vi "I2C_write.vi"(8 "Min time SCL Low":u32 caption="Low", 9 "Min time SCL High":u32 caption="High", 11 "Data":u8[](array[numeric])) -> ()   [LabVIEW 2019]
uses:
  <vilib>/rvi/Emulation/niFpgaGetClockAttributes.vi
  <vilib>/rvi/Emulation/niFpgaSctlEmulationGetInTimedLoop.vi
  <vilib>/rvi/Emulation/niFpgaEmulationReportErrorSimple.vi
  <vilib>/rvi/eio/common/nirviEmuTemplateMethod_errors.vi
  <vilib>/rvi/Emulation/niFpgaCriticalErrorInLSC.vi
  <vilib>/eio/EIONode/EIONode.xnode
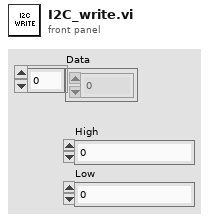
[diagram p1: front panel]
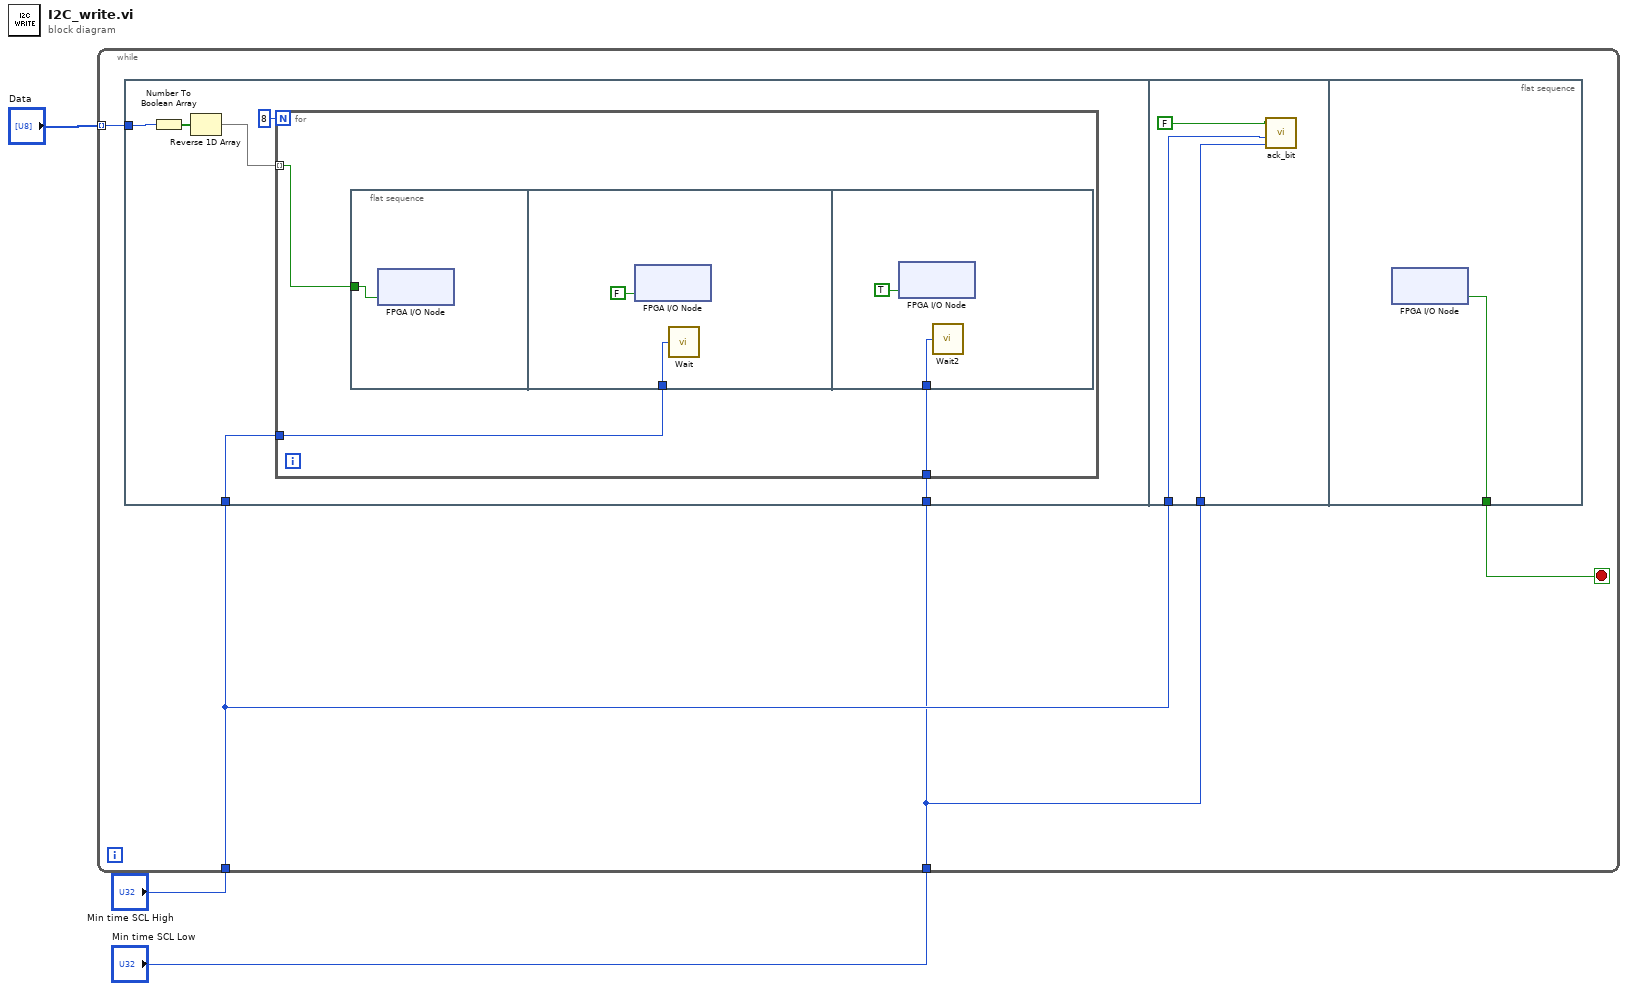
[diagram p0: block diagram]
diagram:
  n1 = while {
    tunnel: "Min time SCL High" -> [w7]
    tunnel: "Min time SCL Low" -> [w6]
    tunnel: "Data" -> [w5] mode=indexing
    stop <- w4 stop-if-true
    n2 = flat-sequence {
      tunnel: w5 -> [w8]
      tunnel: w7 -> [w10]
      tunnel: w6 -> [w9]
      tunnel: w7 -> [w23]
      tunnel: w6 -> [w22]
      tunnel: [w25] -> w4
      frame #0 {
        n3 = Number To Boolean Array(number=w8) -> (Boolean array=w13:bool[])
        n4 = Reverse 1D Array(array=w13) -> (reversed array=w11:bool[])
        n5 = for {
          N: 8 -> [_]
          tunnel: w11 -> [w16] mode=indexing
          tunnel: w10 -> [w15]
          tunnel: w9 -> [w14]
          n6 = flat-sequence {
            tunnel: w16 -> [w17]
            tunnel: w15 -> [w18]
            tunnel: w14 -> [w20]
            frame #0 {
              n7 = xnode "FPGA I/O Node"("SDA"=w17) -> ()  [unwired: 1 in, 1 out]
            }
            frame #1 {
              n8 = xnode "FPGA I/O Node"("SCL"=FALSE ("ConnectorA/DIO14")) -> ()  [unwired: 1 in, 1 out]
              n9 = call "Wait"("Count(uSec)"=w18) -> ()  [unwired: 1 out]
            }
            frame #2 {
              n10 = xnode "FPGA I/O Node"("SCL"=TRUE ("ConnectorA/DIO14")) -> ()  [unwired: 1 in, 1 out]
              n11 = call "Wait2"("Count(uSec)"=w20) -> ()  [unwired: 1 out]
            }
          }
        }
      }
      frame #1 {
        n12 = call "ack_bit.vi"("Min time SCL Low"=w22, "Min Time SCL High"=w23, "ack"=FALSE ("Acknowledgement")) -> ()  [unwired: 9 in]
      }
      frame #2 {
        n13 = xnode "FPGA I/O Node"() -> ("SDA"=w25:bool)  [unwired: 1 in, 1 out]
      }
    }
  }
